vi "Long_Pause_Press_Stop.vi"(8 "error in (no error)":errorcluster) -> (0 "error out":errorcluster, 3 "Stop":bool)   [LabVIEW 2014]
uses:
  <userlib>/UCSD Robotics Lab/Robotics-Cape/LV/libroboticscape.lvlib
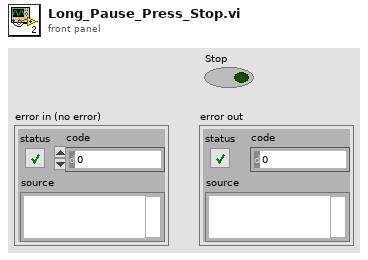
[diagram p1: front panel]
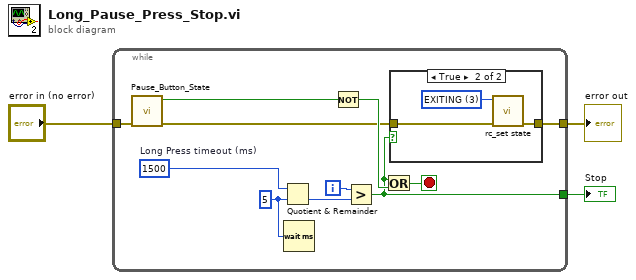
[diagram p0: block diagram]
diagram:
  n1 = while {
    tunnel: "error in (no error)" -> [w13]
    tunnel: [w5] -> w2
    tunnel: [w4] -> w3
    i -> [w14]
    stop <- w11 stop-if-true
    w10 = 1500  # Long Press timeout (ms)
    w7 = u32 5 ("milliseconds to wait")
    n2 = call "Pause_Button_State.vi"("error in (no error)"=w13) -> ("error out"=w6:errorcluster, "Boolean"=w12:bool)  [unwired: 9 in]
    n3 = Quotient & Remainder(x=w10, y=w7) -> (floor(x/y)=w9:u32)  [unwired: 1 out]
    n4 = Wait (ms)(milliseconds to wait=w7) -> ()  [unwired: 1 out]
    n5 = Not(x=w12) -> (.not. x?=w8:bool)
    n6 = Greater?(x=w14, y=w9) -> (0:w4:bool)
    n7 = Or(x=w4, y=w8) -> (x .or. y?=w11:bool)
    n8 = case shown="True" w4 {
      tunnel: w6 -> [w15 w18]
      tunnel: [w15 w17] -> w5
      frame False {
      }
      frame True {
        w16 = u32 3 items=["UNINITIALIZED", "RUNNING", "PAUSED", "EXITING"] ("new_state")
        n9 = call <userlib>:"rc_set state.vi"("error in (no error)"=w18, "new_state"=w16) -> ("error out"=w17:errorcluster)  [unwired: 8 in, 1 out]
      }
    }
  }
  "Stop" <- w3
  "error out" <- w2
